vi "CF_Z_Bridge_to_DSC.vi"(0 "description, string":refnum<k21>="ni.var.psp://housesoftheholy/Leiden CF900/CF_TC_Z_description", 1 "dbl var":refnum<k21>[](array[refnum])=["ni.var.psp://housesoftheholy/Leiden CF900/CF_TC_Z_R0", "ni.var.psp://housesoftheholy/Leiden CF900/CF_TC_Z_R1", "ni.var.psp://housesoftheholy/Leiden CF900/CF_TC_Z_R2", "ni.var.psp://housesoftheholy/Leiden CF900/CF_TC_Z_R3", "ni.var.psp://housesoftheholy/Leiden CF900/CF_TC_Z_R4", "ni.var.psp://housesoftheholy/Leiden CF900/CF_TC_Z_R5", "ni.var.psp://housesoftheholy/Leiden CF900/CF_TC_Z_R6", "ni.var.psp://housesoftheholy/Leiden CF900/CF_TC_Z_R7", "ni.var.psp://housesoftheholy/Leiden CF900/CF_TC_Z_R8", "ni.var.psp://housesoftheholy/Leiden CF900/CF_TC_Z_R9", "ni.var.psp://housesoftheholy/Leiden CF900/CF_TC_Z_T0", "ni.var.psp://housesoftheholy/Leiden CF900/CF_TC_Z_T1", "ni.var.psp://housesoftheholy/Leiden CF900/CF_TC_Z_T2", "ni.var.psp://housesoftheholy/Leiden CF900/CF_TC_Z_T3", "ni.var.psp://housesoftheholy/Leiden CF900/CF_TC_Z_T4", "ni.var.psp://housesoftheholy/Leiden CF900/CF_TC_Z_T5", "ni.var.psp://housesoftheholy/Leiden CF900/CF_TC_Z_T6", "ni.var.psp://housesoftheholy/Leiden CF900/CF_TC_Z_T7", "ni.var.psp://housesoftheholy/Leiden CF900/CF_TC_Z_T8", "ni.var.psp://housesoftheholy/Leiden CF900/CF_TC_Z_T9"], 2 "dbl":dbl[](array[numeric])=[-1e+30, 3977.4776241280374, 3649.809852131724, 0.0, 17313.58847758918, 0.0, 0.0, 0.0, 0.0, 0.0, -5.724e-36, 4025.436136585684, 4054.3239935153424, nan, 4258.3107502810735, 0.0, 0.0, 0.0, 0.0, 0.0], 5 "String In":string="3K, Still, 50 mK, MC, MC, , , , , ", 7 "calibration string":refnum<k21>="ni.var.psp://housesoftheholy/Leiden CF900/CF_TC_Z_calibration", 9 "String In 2":string="CMN 187_TC_2-29, 140701_OuterSP (fit from fit, self defined fx)_TC, 140702_Solenoid (Right, fit from fit, self defined fx)_TC, RuO2_10K_TC, RuO2_10K_TC, No Calibration, No Calibration, No Calibration, No Calibration, No Calibration", 11 "error in (no error)":errorcluster) -> (15 "error out":errorcluster)   [LabVIEW 2013]
panel:
  # "CF Impedence Bridge to DSC"
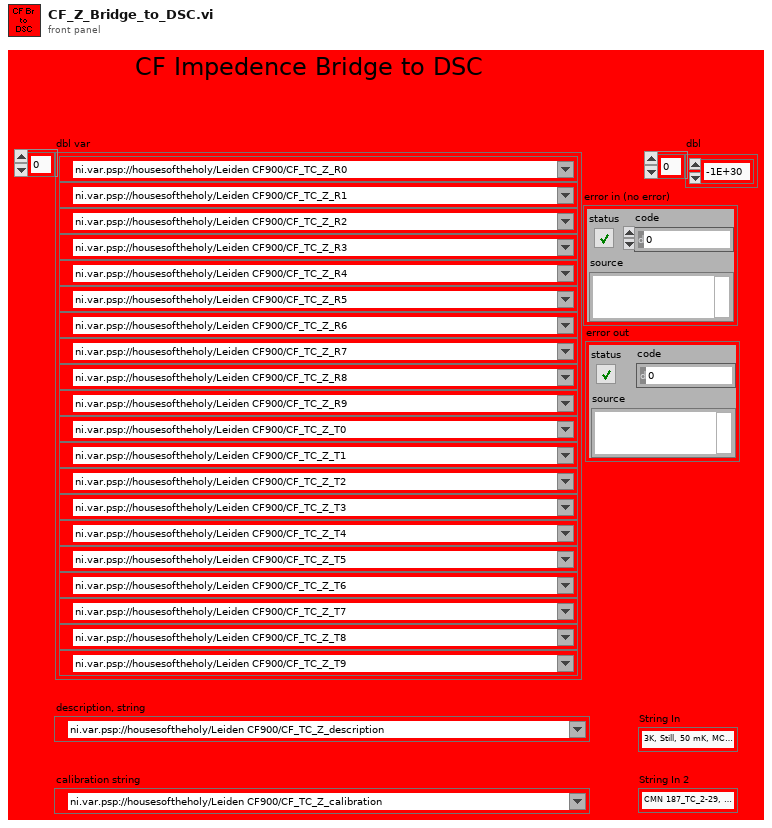
[diagram p1: front panel]
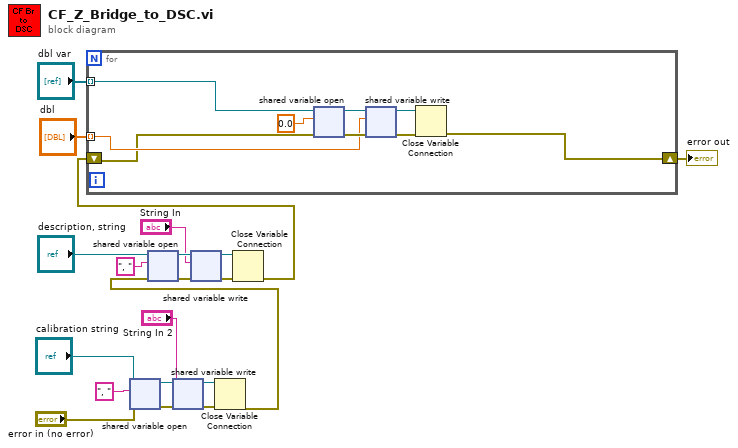
[diagram p0: block diagram]
diagram:
  n1 = shared-variable-open("calibration string", "error in (no error)", ", " ("string")) -> (w10:refnum<k21>, w9:errorcluster)  [unwired: 1 in]
  n2 = shared-variable-write(w10, w9, "String In 2") -> (w11:refnum<k21>, w8:errorcluster)
  n3 = Close Variable Connection(8:w8, 11:w11) -> (0:w3:errorcluster)
  n4 = shared-variable-open("description, string", w3, ", " ("string")) -> (w17:refnum<k21>, w16:errorcluster)  [unwired: 1 in]
  n5 = shared-variable-write(w17, w16, "String In") -> (w18:refnum<k21>, w15:errorcluster)
  n6 = Close Variable Connection(8:w15, 11:w18) -> (0:w4:errorcluster)
  n7 = for {
    tunnel: "dbl var" -> [w24] mode=indexing
    tunnel: "dbl" -> [w23] mode=indexing
    shift-right: [w22] -> w1
    shift-left: w4 -> [w21]
    n8 = shared-variable-open(w24, w21, 0.0) -> (w27:refnum<k21>, w28:errorcluster)  [unwired: 1 in]
    n9 = shared-variable-write(w27, w28, w23) -> (w26:refnum<k21>, w29:errorcluster)
    n10 = Close Variable Connection(8:w29, 11:w26) -> (0:w22:errorcluster)
  }
  "error out" <- w1
